vi "Setup DI.vi"(0 "reference in":refnum<class "DI.lvclass">, 2 "Module Names (NI-MAX Alias)":string[](array[string])=["DI-Sink-32CH-1", "DI-Sink-32CH-2"], 3 "DAQ Port Number":u32, 4 "Number of Channels Per Module":u32[](array[numeric])=[32, 32], 5 "error in (no error)":errorcluster) -> (14 "reference out":refnum<class "DI.lvclass">, 19 "error out":errorcluster)   [LabVIEW 2017, in "DI.lvclass"]
uses:
  DI.lvclass
  <vilib>/DAQmx/create/channels.llb/DAQmx Create Channel (DI-Digital Input).vi
  <resource>/objmgr/daqmx.rc
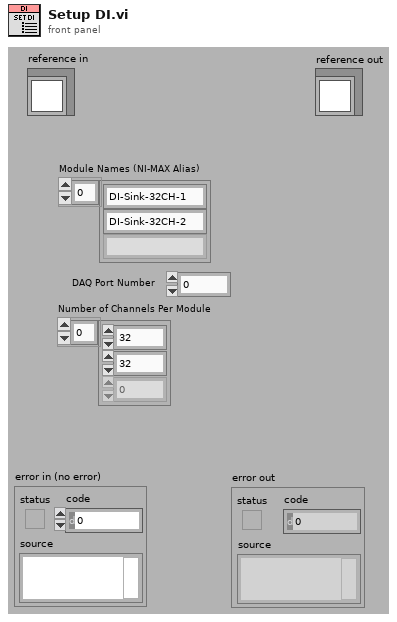
[diagram p1: front panel]
types:
  T1 = typedef "DI.lvclass/ObjectAttributes.ctl" = cluster{"DI Task":refnum<k21>, "DI Status":bool[], "DI Module Names (NI-Max Name)":string[], "Number of Channels Per DI Module":i32[], "Number of DI Modules":u32, "Number of Total DI Channels":u32, "DI On/Off Status":bool, "DO VI Reference":refnum<vi>}
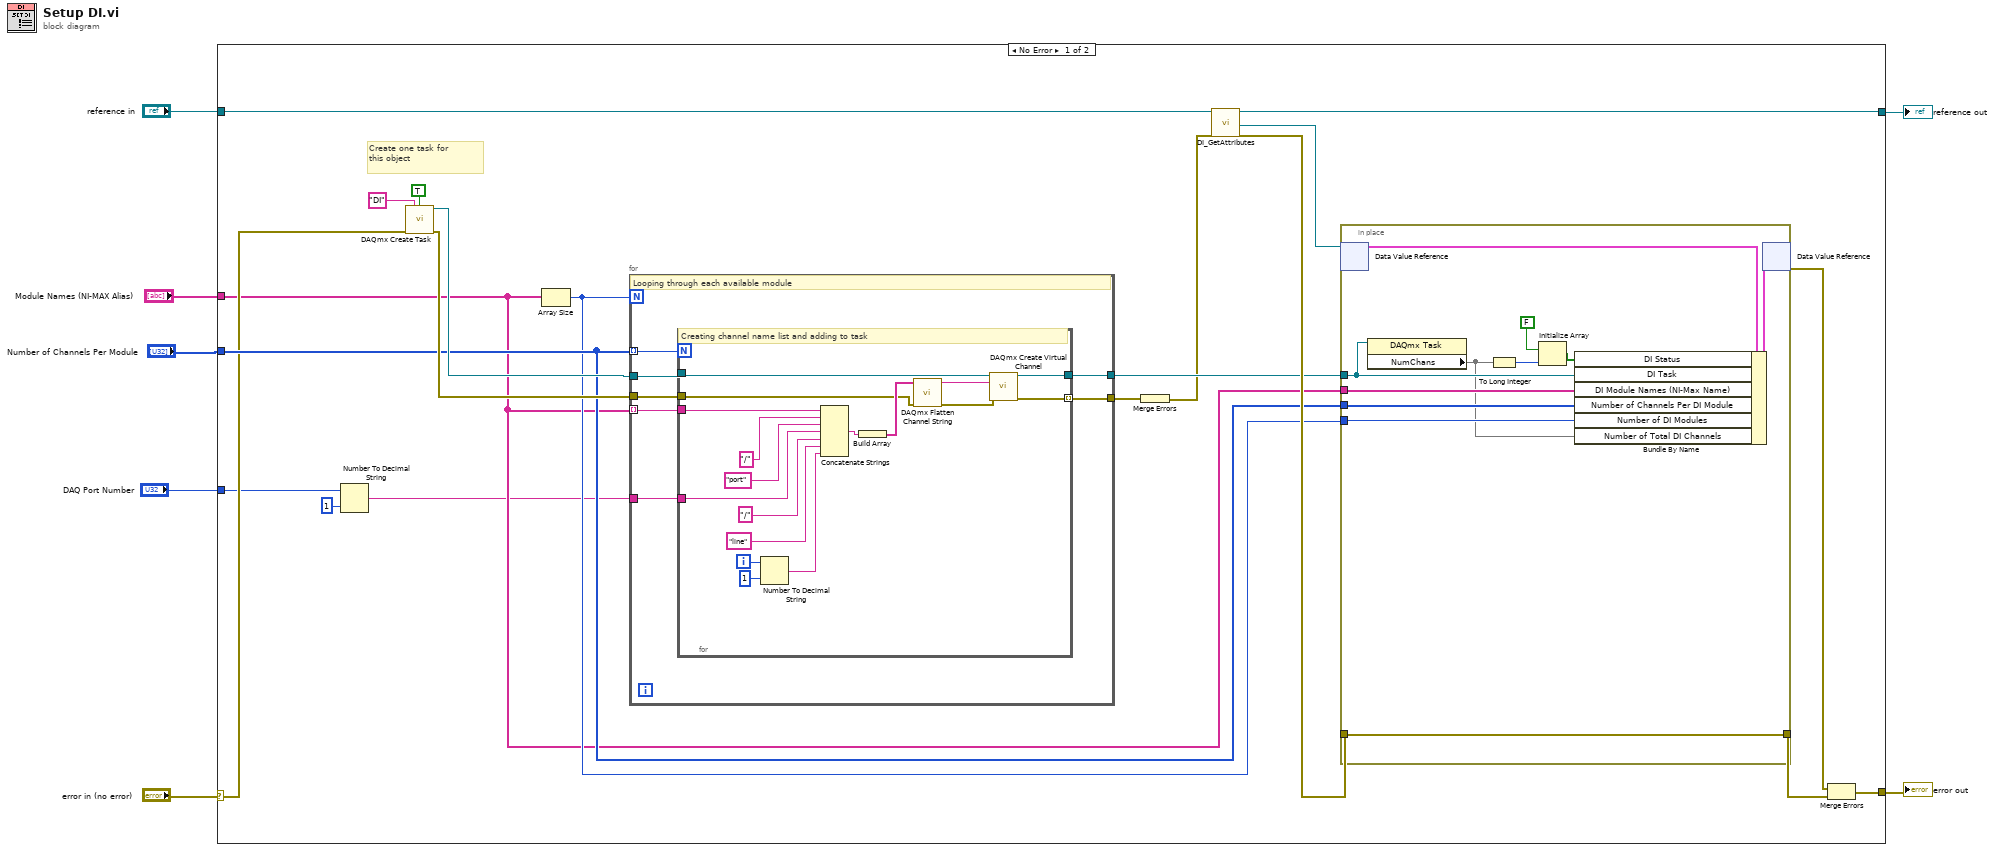
[diagram p0: block diagram]
diagram:
  n1 = case shown="No Error" "error in (no error)" {
    selector: "error in (no error)" -> [w13 w65]
    tunnel: [w25 w65] -> w6
    tunnel: [w26 w64] -> w4
    tunnel: "reference in" -> [w28 w64]
    tunnel: "Module Names (NI-MAX Alias)" -> [w12 _]
    tunnel: "Number of Channels Per Module" -> [w15 _]
    tunnel: "DAQ Port Number" -> [w9 _]
    frame No Error {
      # "Create one task for \nthis object"
      n2 = Number To Decimal String(number=w9, width (-)=i16 1) -> (decimal integer string=w8:string)
      n3 = call <vilib>:"DAQmx Create Task.vi"("new task name"="DI", "auto cleanup"=TRUE, "error in"=w13) -> ("task out"=w19:refnum<k21>, "error out"=w21:errorcluster)  [unwired: 11 in]
      n4 = Array Size(array=w12) -> (size(s)=w14:i32)
      n5 = for {
        N: w14 -> [_]
        tunnel: w21 -> [w46]
        tunnel: [w45] -> w17
        tunnel: w15 -> [w44] mode=indexing
        tunnel: w19 -> [w43]
        tunnel: [w42] -> w18
        tunnel: w12 -> [w41] mode=indexing
        tunnel: w8 -> [w40]
        # "Looping through each available module"
        n6 = for {
          N: w44 -> [_]
          tunnel: w43 -> [w59]
          tunnel: [w58] -> w42
          tunnel: w46 -> [w54]
          tunnel: [w53] -> w45 mode=indexing
          tunnel: w41 -> [w51]
          tunnel: w40 -> [w50]
          i -> [w52]
          # "Creating channel name list and adding to task"
          n7 = Number To Decimal String(number=w52, width (-)=i16 1) -> (decimal integer string=w47:string)
          n8 = Concatenate Strings(w51, "/", "port", w50, "/", "line", w47) -> (w57:string)
          n9 = Build Array(w57) -> (w56:string[])
          n10 = call <vilib>:"DAQmx Flatten Channel String.vi"("names in"=w56, "error in"=w54) -> ("names out"=w60:string, "error out"=w61:errorcluster)  [unwired: 12 in]
          n11 = call-poly <vilib>:"DAQmx Create Virtual Channel.vi"("task in"=w59, "lines"=w60, "error in"=w61) -> ("task out"=w58:refnum<k21>, "error out"=w53:errorcluster)  [unwired: 11 in]
        }
      }
      n12 = Merge Errors(w17) -> (w16:errorcluster)
      n13 = call "DI_GetAttributes.vi"("reference in"=w28, "error in (no error)"=w16) -> ("reference out"=w26:refnum<class "DI.lvclass">, "DataRef"=w24:refnum<data-value>, "error out"=w23:errorcluster)  [unwired: 14 in, 1 out]
      n14 = in-place {
        in-place-border: w23 -> [w37]
        in-place-border: [w37] -> w22
        in-place-border: w18 -> [w36]
        in-place-border: w12 -> [w33]
        in-place-border: w15 -> [w32]
        in-place-border: w14 -> [w31]
        n15 = in-place-dvr #1(w24) -> (w38:T1)  [unwired: 1 out]
        n16 = property class="DAQmx Task"(reference=w36) -> ("NumChans"=w29)  [unwired: 1 in, 2 out]
        n17 = To Long Integer(number=w29) -> (32bit integer=w30:i32)
        n18 = Initialize Array(FALSE, w30) -> (w34:bool[])
        n19 = Bundle By Name(cluster=w38, "DI Status"=w34, "DI Task"=w36, "DI Module Names (NI-Max Name)"=w33, "Number of Channels Per DI Module"=w32, "Number of DI Modules"=w31, "Number of Total DI Channels"=w29) -> (w39:T1)
        n20 = in-place-dvr #1(w39) -> (w27:errorcluster)  [unwired: 1 out]
      }
      n21 = Merge Errors(w27, w22) -> (w25:errorcluster)
    }
    frame Error {
    }
  }
  "error out" <- w6
  "reference out" <- w4
